vi "DiagnosticsH1R-old.vi"(7 "Intergation time":dbl, 10 "Update previous array?":bool, 11 "Array":dbl[][](array[numeric])) -> (0 "RMS subtr ADU  (raw)":dbl format="%#.2f", 1 "mean subtracted ADU (raw)":dbl format="%#.2f", 2 "Median (ADU/sec)":dbl format="%#_3f", 3 "Histogram Graph":T1(graph))   [LabVIEW 2010]
uses:
  <vilib>/Analysis/NI_AALPro.lvlib
panel:
  out "Median e-/sec":dbl format="%#_3f"
  out "Median e- (raw)":dbl
  in  "e-/ADU":dbl=3.0
  out "Median ADU  raw":dbl
  out "Array previous":dbl[][](array[numeric])
  out "# outside":cluster{"total":i32, "below":i32, "above":i32}
  in  "# bins":i32
  in  "min":dbl format="%0.2f"
  in  "max":dbl format="%0.2f"
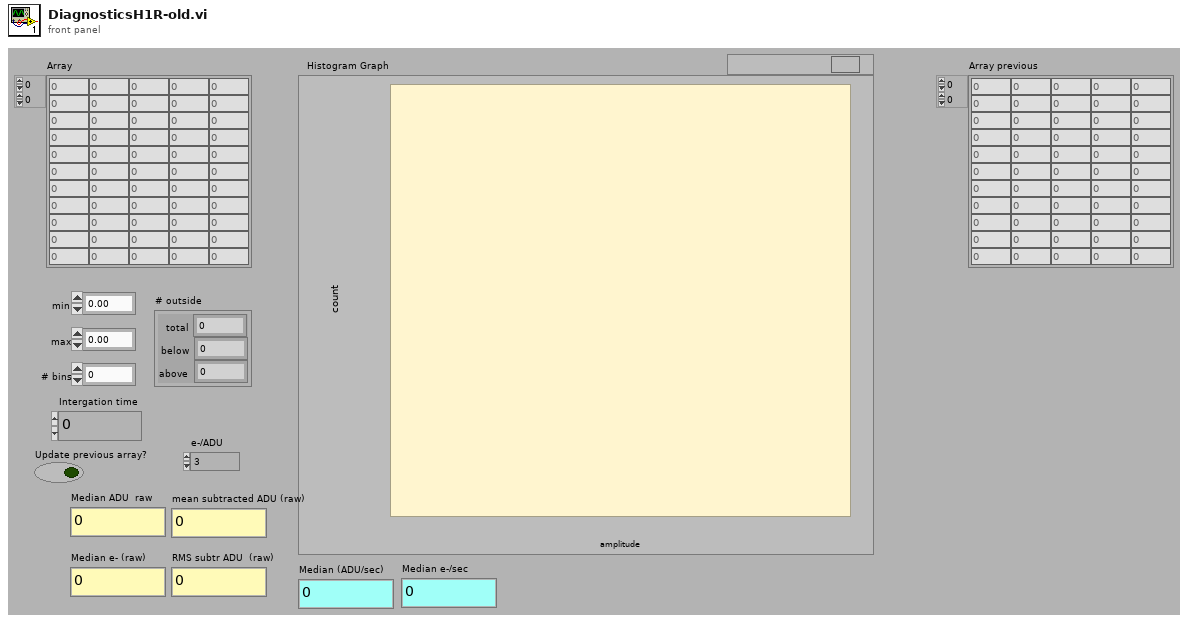
[diagram p1: front panel]
types:
  T1 = cluster{"X Values":dbl[], "Histogram: h(x)":i32[]}
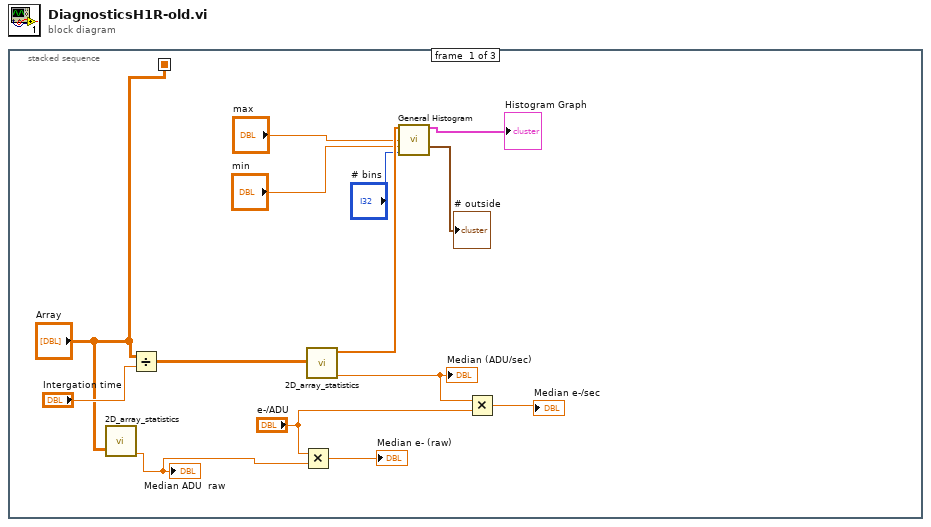
[diagram p0: block diagram]
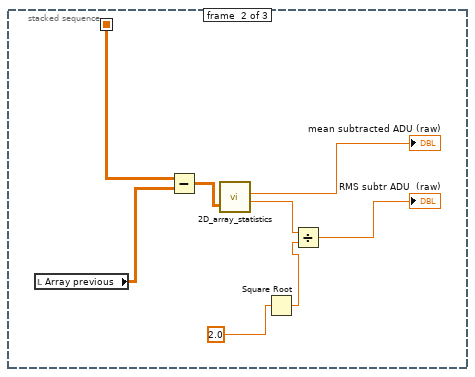
[diagram p2: hidden frame]
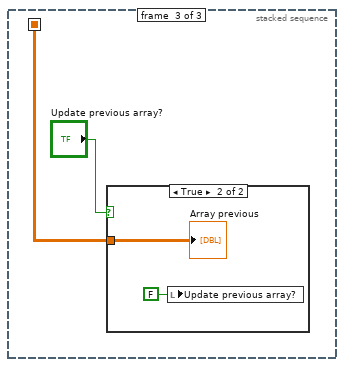
[diagram p3: hidden frame]
diagram:
  n1 = stacked-sequence {
    seq-local: ["Array" _ _] -> [_ w22 w24]
    frame #0 {
      n2 = call "2D_array_statistics.vi"("Array"="Array") -> ("median"=w5:dbl)  [unwired: 2 in, 3 out]
      "Median ADU  raw" <- w5
      n3 = Divide(x="Array", y="Intergation time") -> (x/y=w7:dbl[][])
      n4 = Multiply(x="e-/ADU", y=w5) -> (x*y=→"Median e- (raw)":dbl)
      n5 = call "2D_array_statistics.vi"("Array"=w7) -> ("1D array"=w14:dbl[], "median"=w3:dbl)  [unwired: 2 in, 2 out]
      "Median (ADU/sec)" <- w3
      n6 = call <vilib>:"General Histogram.vi"("X"=w14, "max"="max", "min"="min", "# bins"="# bins") -> ("Histogram Graph"=→"Histogram Graph":T1, "# outside"=→"# outside":cluster{"total":i32, "below":i32, "above":i32})  [unwired: 7 in, 3 out]
      n7 = Multiply(x=w3, y="e-/ADU") -> (x*y=→"Median e-/sec":dbl)
    }
    frame #1 {
      n8 = local read "Array previous"() -> (w21:dbl[][])
      n9 = Subtract(x=w22, y=w21) -> (x-y=w20:dbl[][])
      n10 = call "2D_array_statistics.vi"("Array"=w20) -> ("mean"=→"mean subtracted ADU (raw)":dbl, "RMS"=w17:dbl)  [unwired: 2 in, 2 out]
      n11 = Square Root(x=2.0) -> (sqrt(x)=w16:dbl)
      n12 = Divide(x=w17, y=w16) -> (x/y=→"RMS subtr ADU  (raw)":dbl)
    }
    frame #2 {
      n13 = case shown="True" "Update previous array?" {
        tunnel: w24 -> [_ w26]
        frame False {
        }
        frame True {
          n14 = local write "Update previous array?"(FALSE ("Update previous array?")) -> ()
          "Array previous" <- w26
        }
      }
    }
  }
